vi "Configure AC Filter.vi"(8 "error in (no error)":errorcluster, 10 "AC Filter Bandwidth (20 Hz)":i32(ring)=20 items=["3"=3, "20"=20, "200"=200], 11 "VISA resource name":refnum<visa-resource-name>) -> (0 "error out":errorcluster, 3 "VISA resource name out":refnum<visa-resource-name>)   [LabVIEW 2010, in "Fluke 884X Series.lvlib"]
doc: "Configures the AC Filter to allow better low frequency accuracy or faster AC settling times."
uses:
  <instrlib>/Fluke 884X Series/Fluke 884X Series.lvlib
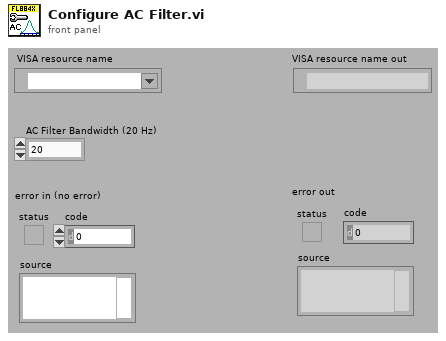
[diagram p1: front panel]
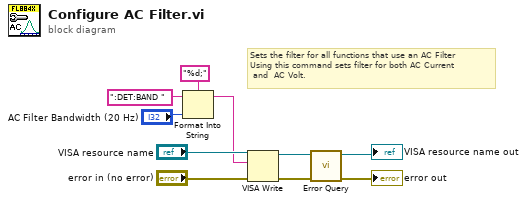
[diagram p0: block diagram]
diagram:
  # "Sets the filter for all functions that use an AC Filter\nUsing this command sets filter for both AC Current\n and  AC Volt."
  n1 = Format Into String(format string="%d;", initial string=":DET:BAND ", "AC Filter Bandwidth (20 Hz)") -> (resulting string=w1:string)  [unwired: 1 in, 1 out]
  n2 = VISA Write(VISA resource name="VISA resource name", write buffer=w1, error in (no error)="error in (no error)") -> (VISA resource name out=w5:refnum<visa-resource-name>, error out=w6:errorcluster)  [unwired: 1 out]
  n3 = call <instrlib>:"Error Query.vi"("error in (no error)"=w6, "VISA resource name"=w5) -> ("error out"=→"error out":errorcluster, "VISA resource name out"=→"VISA resource name out":refnum<visa-resource-name>)  [unwired: 6 in, 2 out]
